vi "Alarm Colors.vi"() -> (2 "Non-critical":u32(colorbox)=16774466, 3 "Critical":u32(colorbox)=16711767)   [LabVIEW 2018, in "Dynamic Shared Variables.lvlib"]
uses:
  Dynamic Shared Variables.lvlib
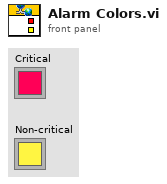
[diagram p1: front panel]
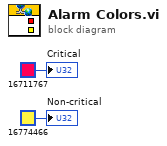
[diagram p0: block diagram]
diagram:
  "Critical" <- u32 16711767
  "Non-critical" <- u32 16774466
